vi "skipMatColRow.vi"(7 "Matrix":dbl[][](array[numeric]), 8 "error in (no error)":errorcluster, 9 "Skip Col Idx":i32[](array[numeric]), 10 "Skip Row Idx":i32[](array[numeric]), 11 "MatOper in":refnum<class "MatOper.lvclass">) -> (0 "error out":errorcluster, 2 "Sub-Array":dbl[][](array[numeric]), 3 "MatOper out":refnum<class "MatOper.lvclass">)   [LabVIEW 2016, in "MatOper.lvclass"]
doc: "Skip the rows or columns in a matrix."
uses:
  MatOper.lvclass
  getSubArray2D.vi
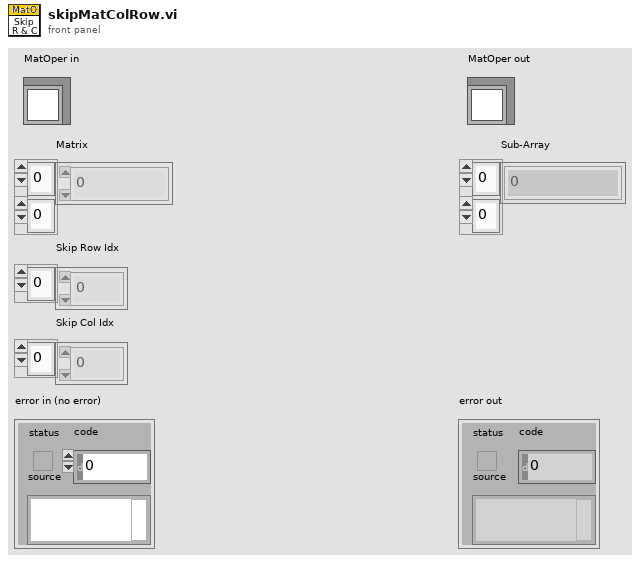
[diagram p1: front panel]
types:
  T1 = cluster{"Non-Overlap Idx Array":i32[], "Non-Overlap Idx Array":i32[]}
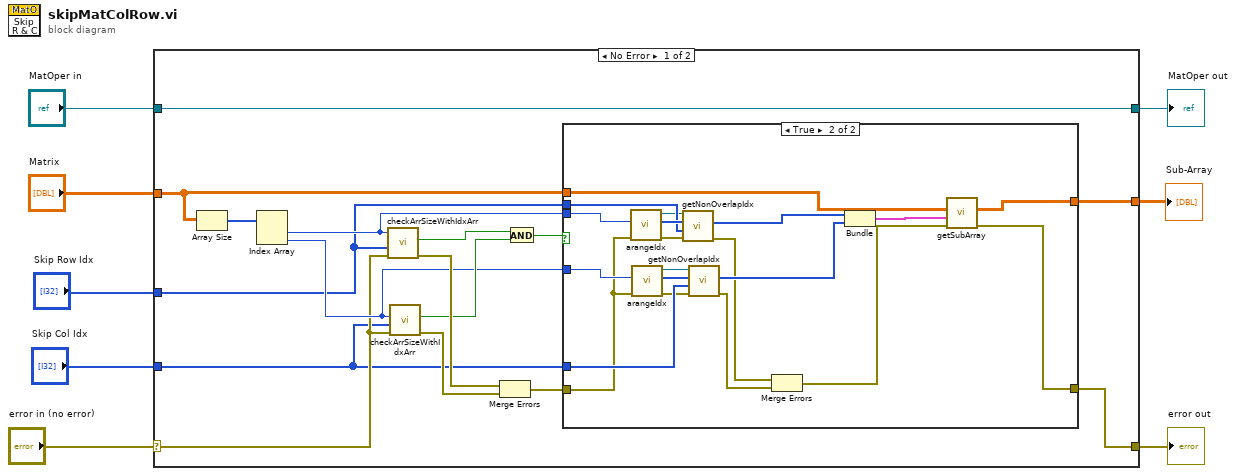
[diagram p0: block diagram]
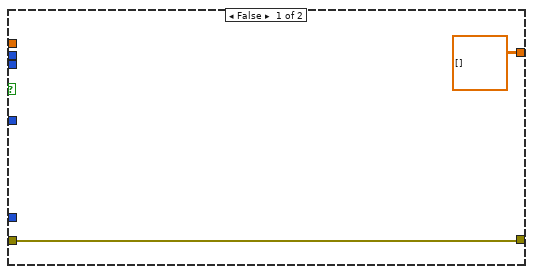
[diagram p2: hidden frame]
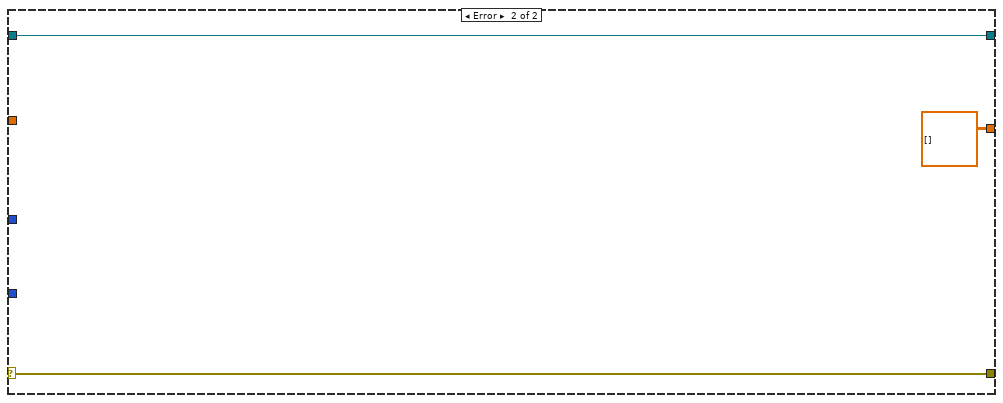
[diagram p3: hidden frame]
diagram:
  n1 = case shown="No Error" "error in (no error)" {
    selector: "error in (no error)" -> [w14 w49]
    tunnel: [w13 w49] -> w7
    tunnel: [w24 w48] -> w5
    tunnel: "MatOper in" -> [w24 w48]
    tunnel: [w12 dbl[][] [] ("Sub-Array")] -> w4
    tunnel: "Matrix" -> [w11 _]
    tunnel: "Skip Row Idx" -> [w10 _]
    tunnel: "Skip Col Idx" -> [w9 _]
    frame No Error {
      n2 = Array Size(array=w11) -> (size(s)=w23:i32[])
      n3 = Index Array(array=w23) -> (element #1=w17:i32, element #2=w16:i32)  [unwired: 2 in]
      n4 = call "checkArrSizeWithIdxArr.vi"("error in (no error)"=w14, "Idx Array"=w10, "Array Size"=w17) -> ("error out"=w22:errorcluster, "In Spec"=w20:bool)  [unwired: 6 in, 1 out]
      n5 = call "checkArrSizeWithIdxArr.vi"("error in (no error)"=w14, "Idx Array"=w9, "Array Size"=w16) -> ("error out"=w21:errorcluster, "In Spec"=w19:bool)  [unwired: 6 in, 1 out]
      n6 = Merge Errors(w22, w21) -> (w15:errorcluster)
      n7 = And(x=w20, y=w19) -> (x .and. y?=w18:bool)
      n8 = case shown="True" w18 {
        tunnel: w17 -> [_ w41]
        tunnel: w16 -> [_ w40]
        tunnel: w15 -> [w25 w30]
        tunnel: w10 -> [_ w39]
        tunnel: w9 -> [_ w38]
        tunnel: w11 -> [_ w37]
        tunnel: [w25 w36] -> w13
        tunnel: [dbl[][] [] ("Sub-Array") w35] -> w12
        frame False {
        }
        frame True {
          n9 = call "arangeIdx.vi"("error in (no error)"=w30, "Number"=w41) -> ("error out"=w32:errorcluster, "Idx Array"=w42:i32[], "MatOper out"=w34:refnum<class "MatOper.lvclass">)  [unwired: 7 in]
          n10 = call "arangeIdx.vi"("error in (no error)"=w30, "Number"=w40) -> ("error out"=w31:errorcluster, "Idx Array"=w43:i32[], "MatOper out"=w33:refnum<class "MatOper.lvclass">)  [unwired: 7 in]
          n11 = call "getNonOverlapIdx.vi"("error in (no error)"=w32, "Overlap Idx Array"=w39, "Input Idx Array"=w42, "MatOper in"=w34) -> ("error out"=w29:errorcluster, "Non-Overlap Idx Array"=w44:i32[])  [unwired: 5 in, 1 out]
          n12 = call "getNonOverlapIdx.vi"("error in (no error)"=w31, "Overlap Idx Array"=w38, "Input Idx Array"=w43, "MatOper in"=w33) -> ("error out"=w28:errorcluster, "Non-Overlap Idx Array"=w45:i32[])  [unwired: 5 in, 1 out]
          n13 = Merge Errors(w29, w28) -> (w27:errorcluster)
          n14 = Bundle("Non-Overlap Idx Array"=w44, "Non-Overlap Idx Array"=w45) -> (w46:T1)  [unwired: 1 in]
          n15 = call-poly "getSubArray.vi"("error in (no error)"=w27, "Index Array Cluster"=w46, "2D Array"=w37) -> ("error out"=w36:errorcluster, "Sub-Array"=w35:dbl[][])  [unwired: 6 in, 1 out]
        }
      }
    }
    frame Error {
    }
  }
  "error out" <- w7
  "MatOper out" <- w5
  "Sub-Array" <- w4
